vi "UDT_admittanceLibrary_AdmittanceFilter.vi"() -> (3 "Unit Test Framework Results":T1)   [LabVIEW 2017]
doc: "Use this template to create a user-defined test VI. Define your test requirements and wire the results to the <b>Result (Test)</b> control. Do not modify the <b>Unit Test Framework Results</b> indicator."
uses:
  <vilib>/utf/common/utf_test_result_troll.ctl
  <vilib>/utf/common/utf_test_result.ctl
  <vilib>/utf/common/utf_test_result_failure.ctl
  <vilib>/utf/common/utf_test_comparison_operators.ctl
  <vilib>/utf/common/utf_vi_tag.ctl
  RT/Admittance Controller/Controls/AdmittanceGains.ctl
  <vilib>/Control Software Solutions Ltd/UTF Helper/SubVIs/UTF Double Equals.vi
  <vilib>/Control Software Solutions Ltd/UTF Helper/SubVIs/UTF Boolean Equals.vi
  <vilib>/Control Software Solutions Ltd/UTF Helper/Unit Test Helper.lvlib
  RT/Admittance Controller/admittanceControllerLibrary.lvlib
  <vilib>/utf/NI_UnitTestFramework.lvlib
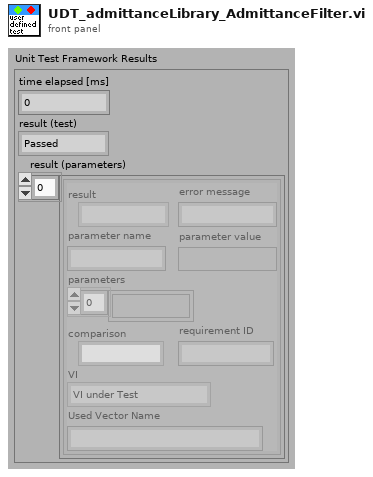
[diagram p1: front panel]
types:
  T1 = typedef "NI_UnitTestFramework.lvlib/utf_test_result_troll.ctl" = cluster{"time elapsed [ms]":u32, "result (test)":T2, "result (parameters)":T3[]}
  T2 = typedef "NI_UnitTestFramework.lvlib/utf_test_result.ctl" = enum16{"Passed", "Failed", "Error", "Skipped", "Not Processed"}
  T3 = typedef "NI_UnitTestFramework.lvlib/utf_test_result_failure.ctl" = cluster{"result":T2, "error message":string, "parameter name":string, "parameter value":variant, "parameters":variant[], "comparison":T4, "requirement ID":string, "VI":T5, "Used Vector Name":string}
  T4 = typedef "NI_UnitTestFramework.lvlib/utf_test_comparison_operators.ctl" = enum16{"=", "!=", ">", ">=", "<", "<=", "range", "symmetric tolerance", "asymmetric tolerance", "string contains", "string not contain", "array size", "string length", "array range", "by element", "array range (limit array)", "user-defined", "array contains", "array not contain", "vector length", "= (elm)", "!= (elm)", "= (case insensitive)", "!= (case insensitive)"}
  T5 = typedef "NI_UnitTestFramework.lvlib/utf_vi_tag.ctl" = enum16{"Setup VI", "VI under Test", "Teardown VI"}
  T6 = typedef "admittanceControllerLibrary.lvlib/AdmittanceGains.ctl" = cluster{"C":dbl, "k":dbl}
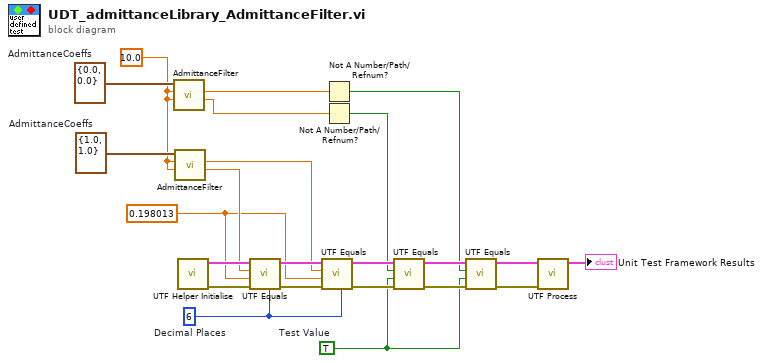
[diagram p0: block diagram]
diagram:
  w1 = TRUE  # Test Value
  w2 = u8 6  # Decimal Places
  w3 = 0.198013
  w10 = 10.0
  w11 = T6 {"C"=1.0, "k"=1.0}  # AdmittanceCoeffs
  w12 = T6 {"C"=0.0, "k"=0.0}  # AdmittanceCoeffs
  n1 = call "AdmittanceFilter.vi"("Fy"=w10, "Fx"=w10, "AdmittanceCoeffs"=w12) -> ("Delta y"=w6:dbl, "Delta x"=w7:dbl)  [unwired: 6 in, 1 out]
  n2 = call "AdmittanceFilter.vi"("Fy"=w10, "Fx"=w10, "AdmittanceCoeffs"=w11) -> ("Delta y"=w9:dbl, "Delta x"=w8:dbl)  [unwired: 6 in, 1 out]
  n3 = call <vilib>:"UTF Helper Initialise.vi"() -> ("error out"=w15:errorcluster, "results array"=w16:T3[])  [unwired: 10 in]
  n4 = call-poly <vilib>:"UTF Equals.vi"("Decimal Places"=w2, "error in (no error)"=w15, "Test Value"=w3, "Input"=w9, "Input Results"=w16) -> ("error out"=w14:errorcluster, "Output Results"=w17:T3[])  [unwired: 5 in]
  n5 = call-poly <vilib>:"UTF Equals.vi"("Decimal Places"=w2, "error in (no error)"=w14, "Test Value"=w3, "Input"=w8, "Input Results"=w17) -> ("error out"=w13:errorcluster, "Output Results"=w18:T3[])  [unwired: 5 in]
  n6 = Not A Number/Path/Refnum?(number/path/refnum=w7) -> (NaN/Path/Refnum?=w4:bool)
  n7 = Not A Number/Path/Refnum?(number/path/refnum=w6) -> (NaN/Path/Refnum?=w5:bool)
  n8 = call-poly <vilib>:"UTF Equals.vi"("error in (no error)"=w13, "Test Value"=w1, "Input"=w5, "Input Results"=w18) -> ("error out"=w22:errorcluster, "Output Results"=w21:T3[])  [unwired: 6 in]
  n9 = call-poly <vilib>:"UTF Equals.vi"("error in (no error)"=w22, "Test Value"=w1, "Input"=w4, "Input Results"=w21) -> ("error out"=w20:errorcluster, "Output Results"=w19:T3[])  [unwired: 6 in]
  n10 = call <vilib>:"UTF Process.vi"("error in (no error)"=w20, "results array"=w19) -> ("Unit Test Framework Results"=→"Unit Test Framework Results":T1)  [unwired: 9 in]
